vi "gRPC Client Test.vi"() -> ()   [LabVIEW 2020, in "FlexLogger_client.lvlib"]
uses:
  FlexLogger_client.lvlib
  RPC Messages/flexlogger_OpenChannelSpecificationDocumentRequest.ctl
  RPC Messages/flexlogger_ProjectIdentifier.ctl
  RPC Messages/flexlogger_SetDataRateLevelRequest.ctl
  RPC Messages/flexlogger_ElementIdentifier.ctl
panel:
  in  "data_rate_level":i32
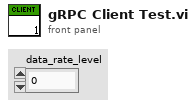
[diagram p1: front panel]
types:
  T1 = typedef "FlexLogger_client.lvlib/flexlogger_OpenChannelSpecificationDocumentRequest.ctl" = cluster{"project":T2}
  T2 = typedef "FlexLogger_client.lvlib/flexlogger_ProjectIdentifier.ctl" = cluster{"project_id":string}
  T3 = typedef "grpc-lvsupport-release.lvlib/grpcId.ctl" = u64
  T4 = typedef "FlexLogger_client.lvlib/flexlogger_GetActiveProjectResponse.ctl" = cluster{"active_project_available":bool, "project":T2}
  T5 = typedef "FlexLogger_client.lvlib/flexlogger_OpenChannelSpecificationDocumentResponse.ctl" = cluster{"document_identifier":T6}
  T6 = typedef "FlexLogger_client.lvlib/flexlogger_ElementIdentifier.ctl" = cluster{"project_id":string, "file_name":string, "element_id":string, "subpart_id":string}
  T7 = typedef "FlexLogger_client.lvlib/flexlogger_GetChannelNamesResponse.ctl" = cluster{"channel_names":string[]}
  T8 = typedef "FlexLogger_client.lvlib/flexlogger_SetDataRateLevelRequest.ctl" = cluster{"document_identifier":T6, "channel_name":string, "data_rate_level":i32}
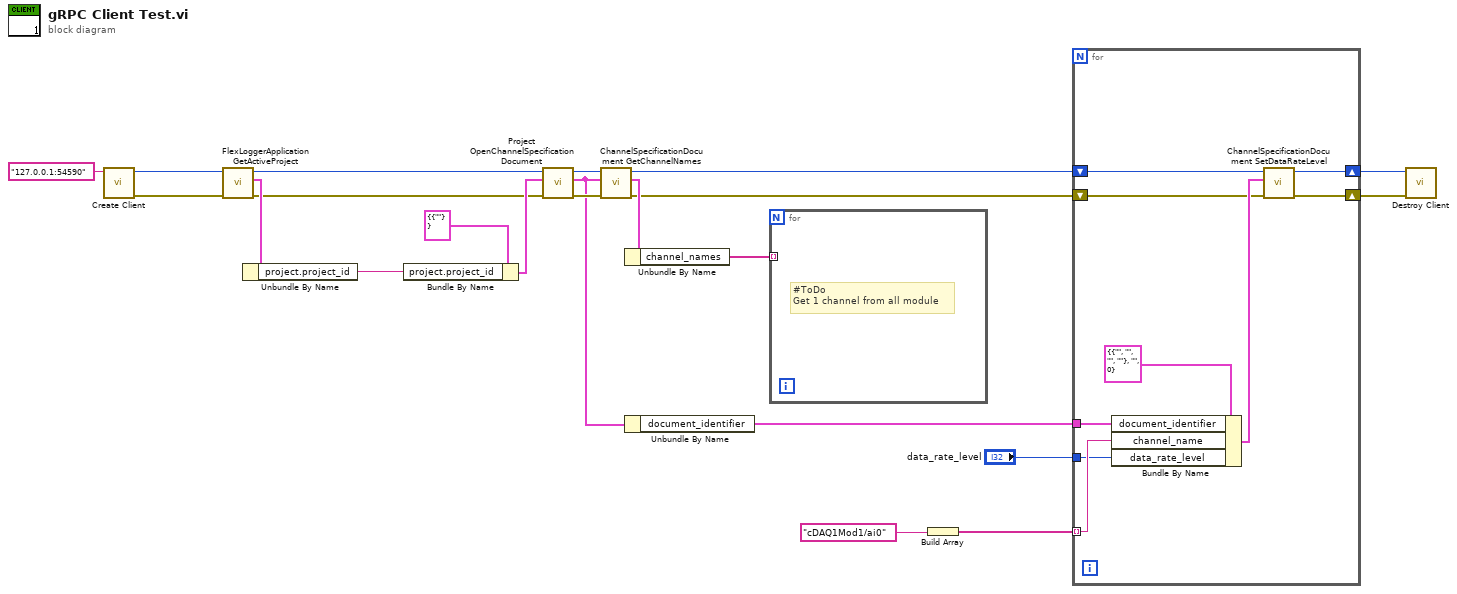
[diagram p0: block diagram]
diagram:
  n1 = call "Create Client.vi"("address"="127.0.0.1:54590") -> ("error out"=w20:errorcluster, "gRPC ID Out"=w21:T3)  [unwired: 9 in]
  n2 = call "FlexLoggerApplication GetActiveProject.vi"("error in"=w20, "gRPC ID"=w21) -> ("error out"=w14:errorcluster, "Response Data"=w19:T4, "gRPC ID out"=w15:T3)  [unwired: 7 in]
  n3 = Unbundle By Name(w19) -> ("project.project_id"=w17:string)
  n4 = Bundle By Name(cluster=T1 {"project"={"project_id"=""}} ("Request Data"), "project.project_id"=w17) -> (w16:T1)
  n5 = call "Project OpenChannelSpecificationDocument.vi"("error in"=w14, "Request Data"=w16, "gRPC ID"=w15) -> ("error out"=w12:errorcluster, "Response Data"=w3:T5, "gRPC ID out"=w13:T3)  [unwired: 6 in]
  n6 = call "ChannelSpecificationDocument GetChannelNames.vi"("error in"=w12, "Request Data"=w3, "gRPC ID"=w13) -> ("error out"=w5:errorcluster, "Response Data"=w11:T7, "gRPC ID out"=w7:T3)  [unwired: 6 in]
  n7 = Unbundle By Name(w11) -> ("channel_names"=w10:string[])
  n8 = Unbundle By Name(w3) -> ("document_identifier"=w2:T6)
  n9 = for {
    tunnel: w10 -> [_] mode=indexing
    # "#ToDo\nGet 1 channel from all module"
  }
  n10 = Build Array("cDAQ1Mod1/ai0") -> (w8:string[])
  n11 = for {
    tunnel: w8 -> [w29] mode=indexing
    shift-right: [w24] -> w6
    shift-left: w7 -> [w26]
    shift-right: [w23] -> w4
    shift-left: w5 -> [w25]
    tunnel: w2 -> [w30]
    tunnel: "data_rate_level" -> [w28]
    n12 = Bundle By Name(cluster=T8 {"document_identifier"={"project_id"="", "file_name"="", "element_id"="", "subpart_id"=""}, "channel_name"="", "data_rate_level"=0} ("Request Data"), "document_identifier"=w30, "channel_name"=w29, "data_rate_level"=w28) -> (w27:T8)
    n13 = call "ChannelSpecificationDocument SetDataRateLevel.vi"("error in"=w25, "Request Data"=w27, "gRPC ID"=w26) -> ("error out"=w23:errorcluster, "gRPC ID out"=w24:T3)  [unwired: 6 in, 1 out]
  }
  n14 = call "Destroy Client.vi"("error in"=w4, "gRPC ID"=w6) -> ()  [unwired: 9 in, 1 out]
